vi "Fetch Waveform Measurement (Time).vi"(0 "VISA resource name":refnum<visa-resource-name>, 5 "Channel A (0:Channel 1)":u16(ring) items=["Channel 1", "Channel 2", "Channel 3", "Channel 4", "Math 1", "Math 2", "Math 3", "Math 4", "Reference 1", "Reference 2", "Reference 3", "Reference 4"], 7 "Function (0:Rise Time)":u16(ring) items=["Rise Time", "Pos Width", "Period", "Fall Time", "Neg Width", "Freq", "+Duty Cycle", "-Duty Cycle", "Delay"], 9 "Channel B (1:Channel 2)":u16(ring)=1 items=["Channel 1", "Channel 2", "Channel 3", "Channel 4", "Math 1", "Math 2", "Math 3", "Math 4", "Reference 1", "Reference 2", "Reference 3", "Reference4"], 11 "error in (no error)":errorcluster, 12 "Search Direction (0:Forward)":u16(ring) items=["Forward", "Backwards"], 13 "Delay Edge1 (0:Rise Time)":u16(ring) items=["Rise Time", "Fall Time "], 14 "Delay Edge2 (0:Rise Time)":u16(ring) items=["Rise Time", "Fall Time"]) -> (4 "VISA resource name out":refnum<visa-resource-name>, 6 "Measurement":dbl, 15 "error out":errorcluster)   [LabVIEW 2011, in "Tektronix 7000 Series.lvlib"]
doc: "Initiates a waveform acquisition on the specified channels and returns a <B>Measurement</B> value. Use the Fetch Waveform Measurement VI separately for any other waveform measurement on a channel without initiating another acquisition."
uses:
  Tektronix 7000 Series.lvlib
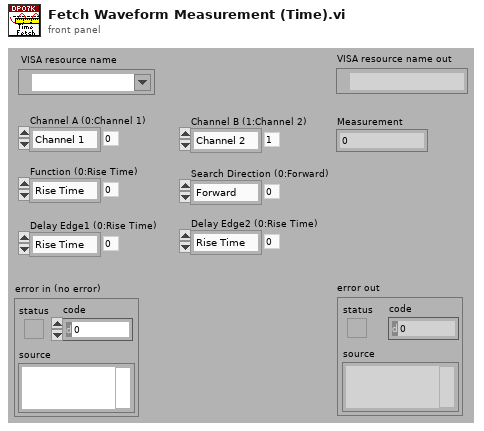
[diagram p1: front panel]
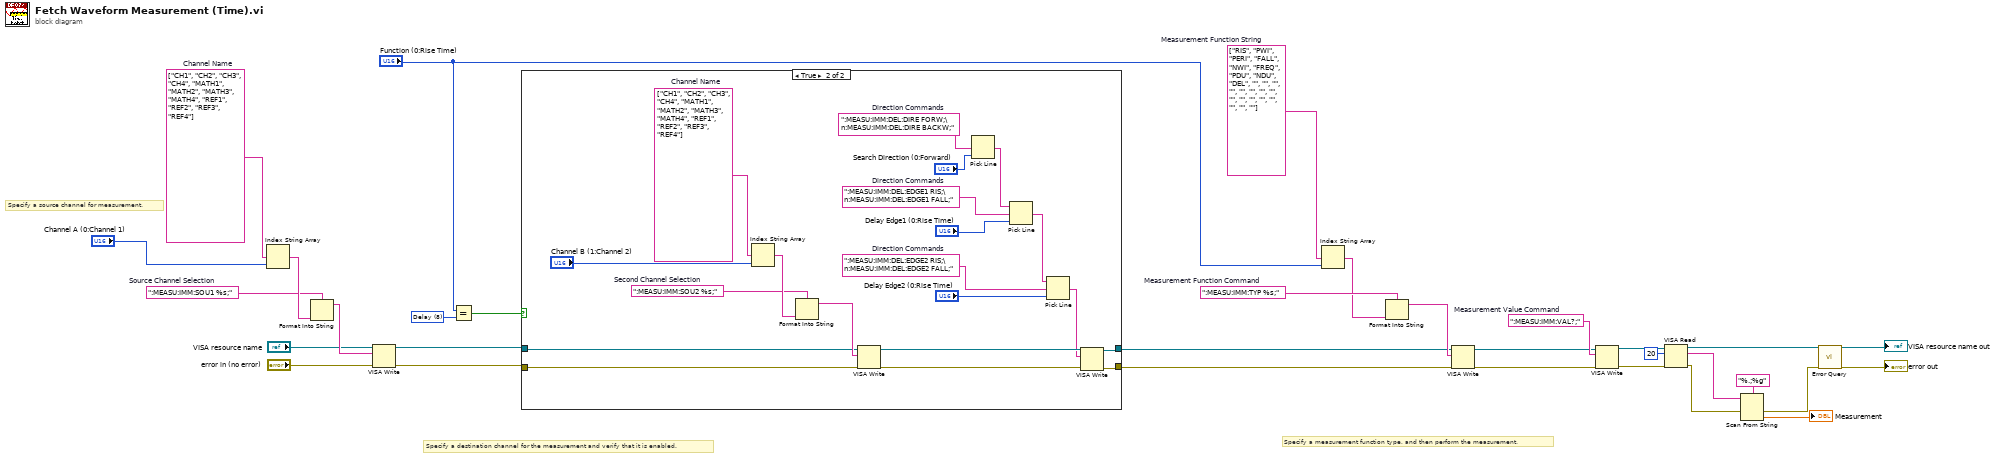
[diagram p0: block diagram]
diagram:
  w9 = u16 8 items=["Rise Time", "Pos Width", "Period", "Fall Time", "Neg Width", "Freq", "+Duty Cycle", "-Duty Cycle", "Delay"] ("Function (0:Raise Time)")
  w11 = string[] ["CH1", "CH2", "CH3", "CH4", "MATH1", "MATH2", "MATH3", "MATH4", "REF1", "REF2", "REF3", "REF4"]  # Channel Name
  w14 = ":MEASU:IMM:SOU1 %s;"  # Source Channel Selection
  w26 = ":MEASU:IMM:VAL?;"  # Measurement Value Command
  w31 = ":MEASU:IMM:TYP %s;"  # Measurement Function Command
  w32 = string[] ["RIS", "PWI", "PERI", "FALL", "NWI", "FREQ", "PDU", "NDU", "DEL", "", "", "", "", "", "", "", "", "", "", "", "", "", "", "", ""]  # Measurement Function String
  # "Specify a source channel for measurement."
  # "Specify a measurement function type, and then perform the measurement."
  # "Specify a destination channel for the measurement and verify that it is enabled."
  n1 = Index String Array(1:"Channel A (0:Channel 1)", 2:w11) -> (0:w15:string)  [unwired: 1 in]
  n2 = Format Into String(format string=w14, w15) -> (resulting string=w13:string)  [unwired: 2 in, 1 out]
  n3 = VISA Write(VISA resource name="VISA resource name", write buffer=w13, error in (no error)="error in (no error)") -> (VISA resource name out=w17:refnum<visa-resource-name>, error out=w16:errorcluster)  [unwired: 1 out]
  n4 = Equal?(x="Function (0:Rise Time)", y=w9) -> (x = y?=w8:bool)
  n5 = case shown="True" w8 {
    tunnel: w17 -> [w34 w36]
    tunnel: w16 -> [w33 w35]
    tunnel: [w34 w41] -> w28
    tunnel: [w33 w40] -> w27
    frame False {
    }
    frame True {
      w51 = string[] ["CH1", "CH2", "CH3", "CH4", "MATH1", "MATH2", "MATH3", "MATH4", "REF1", "REF2", "REF3", "REF4"]  # Channel Name
      w43 = ":MEASU:IMM:DEL:EDGE2 RIS;\n:MEASU:IMM:DEL:EDGE2 FALL;"  # Direction Commands
      w46 = ":MEASU:IMM:DEL:EDGE1 RIS;\n:MEASU:IMM:DEL:EDGE1 FALL;"  # Direction Commands
      w49 = ":MEASU:IMM:DEL:DIRE FORW;\n:MEASU:IMM:DEL:DIRE BACKW;"  # Direction Commands
      w53 = ":MEASU:IMM:SOU2 %s;"  # Second Channel Selection
      n6 = Index String Array(1:"Channel B (1:Channel 2)", 2:w51) -> (0:w54:string)  [unwired: 1 in]
      n7 = Format Into String(format string=w53, w54) -> (resulting string=w52:string)  [unwired: 2 in, 1 out]
      n8 = VISA Write(VISA resource name=w36, write buffer=w52, error in (no error)=w35) -> (VISA resource name out=w39:refnum<visa-resource-name>, error out=w38:errorcluster)  [unwired: 1 out]
      n9 = Pick Line(multi-line string=w49, line index="Search Direction (0:Forward)") -> (output string=w47:string)  [unwired: 1 in]
      n10 = Pick Line(string ("")=w47, multi-line string=w46, line index="Delay Edge1 (0:Rise Time)") -> (output string=w44:string)
      n11 = Pick Line(string ("")=w44, multi-line string=w43, line index="Delay Edge2 (0:Rise Time)") -> (output string=w37:string)
      n12 = VISA Write(VISA resource name=w39, write buffer=w37, error in (no error)=w38) -> (VISA resource name out=w41:refnum<visa-resource-name>, error out=w40:errorcluster)  [unwired: 1 out]
    }
  }
  n13 = Index String Array(1:"Function (0:Rise Time)", 2:w32) -> (0:w30:string)  [unwired: 1 in]
  n14 = Format Into String(format string=w31, w30) -> (resulting string=w29:string)  [unwired: 2 in, 1 out]
  n15 = VISA Write(VISA resource name=w28, write buffer=w29, error in (no error)=w27) -> (VISA resource name out=w19:refnum<visa-resource-name>, error out=w18:errorcluster)  [unwired: 1 out]
  n16 = VISA Write(VISA resource name=w19, write buffer=w26, error in (no error)=w18) -> (VISA resource name out=w25:refnum<visa-resource-name>, error out=w24:errorcluster)  [unwired: 1 out]
  n17 = VISA Read(VISA resource name=w25, byte count=u32 20, error in (no error)=w24) -> (VISA resource name out=w5:refnum<visa-resource-name>, read buffer=w22:string, error out=w4:errorcluster)  [unwired: 1 out]
  n18 = Scan From String(format string="%.;%g", input string=w22, error in=w4) -> (error out=w3:errorcluster, output 1=→"Measurement":dbl)  [unwired: 2 in, 2 out]
  n19 = call "Error Query.vi"("error in (no error)"=w3, "VISA resource name"=w5) -> ("error out"=→"error out":errorcluster, "VISA resource name out"=→"VISA resource name out":refnum<visa-resource-name>)  [unwired: 6 in, 2 out]
